vi "Demo.vi"() -> ()   [LabVIEW 2018]
panel:
  in  "Boolean 41":bool
  in  "Boolean 40":bool
  in  "Boolean 39":bool
  in  "Boolean 38":bool
  in  "Boolean 37":bool
  in  "Boolean 36":bool
  in  "Boolean 35":bool
  in  "Boolean 34":bool
  in  "Boolean 33":bool
  in  "Boolean 32":bool
  in  "Boolean 31":bool
  in  "Boolean 30":bool
  in  "Boolean 29":bool
  in  "Boolean 28":bool
  in  "Boolean 27":bool
  in  "Boolean 26":bool
  in  "Boolean 25":bool
  in  "Boolean 24":bool
  in  "Boolean 23":bool
  in  "Boolean 22":bool
  in  "Boolean 21":bool
  in  "Boolean 20":bool
  in  "Boolean 19":bool
  in  "Boolean 18":bool
  in  "Boolean 17":bool
  in  "Boolean 16":bool
  in  "Boolean 15":bool
  in  "Boolean 14":bool
  in  "Boolean 13":bool
  in  "Boolean 12":bool
  in  "Boolean 11":bool
  in  "Boolean 10":bool
  in  "Boolean 9":bool
  in  "Boolean 8":bool
  in  "Boolean 7":bool
  in  "Boolean 6":bool
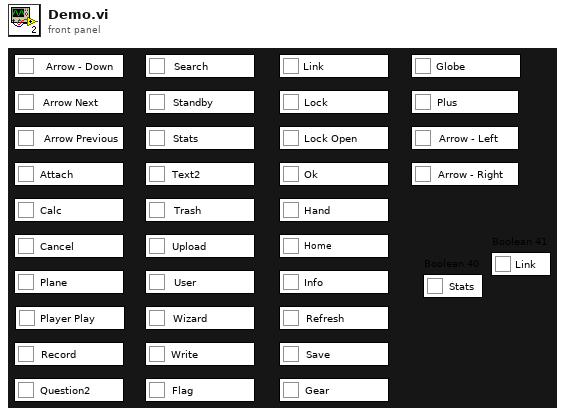
[diagram p1: front panel]
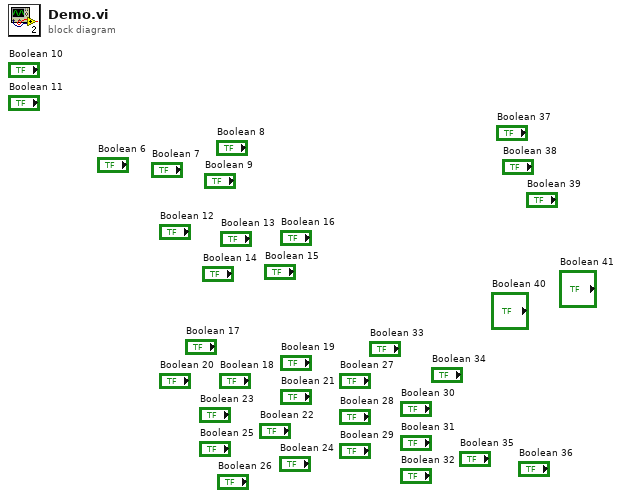
[diagram p0: block diagram]
diagram:
